vi "Initialize.vi"(7 "not in use":string="Setpoint.ch%d.SP", 8 "error in":errorcluster, 9 "Number of Channels":u32=1, 10 "Instance Name":string, 11 "Voltage Actual Value in":refnum<class "Voltage Actual Value.lvclass">) -> (0 "error out":errorcluster, 3 "Voltage Actual Value out":refnum<class "Voltage Actual Value.lvclass">)   [LabVIEW 2023, in "Voltage Actual Value.lvclass"]
uses:
  Voltage Actual Value.lvclass
  Actual Value/Actual Value.lvclass
  Voltage Actual Value.lvclass/Voltage Actual Value.ctl
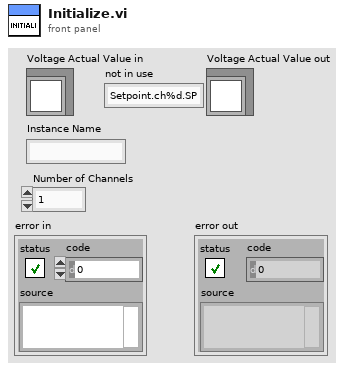
[diagram p1: front panel]
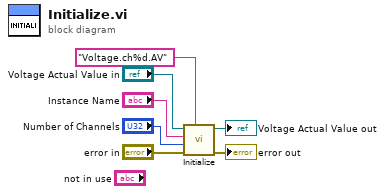
[diagram p0: block diagram]
diagram:
  n1 = call-parent "Initialize.vi"("ChannelName"="Voltage.ch%d.AV", "error in"="error in", "Number of Channels"="Number of Channels", "Instance Name"="Instance Name", "Actual Value in"="Voltage Actual Value in") -> ("error out"=→"error out":errorcluster, "Actual Value out"=→"Voltage Actual Value out":refnum<class "Voltage Actual Value.lvclass">)  [unwired: 5 in]
